vi "USUARIO_CONTRASENA.vi"(9 "INGRESAR (ENTER)":bool, 10 "Clave":string, 11 "Nombre":string) -> (1 "String 2":string, 2 "ACCESO":bool)   [LabVIEW 2019, in "HMI Class 3.lvclass"]
uses:
  HMI Class 3.lvclass
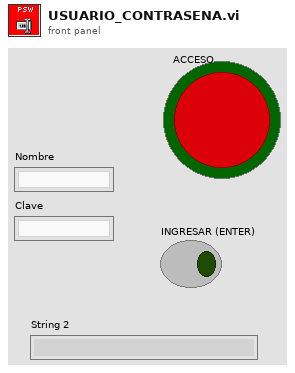
[diagram p1: front panel]
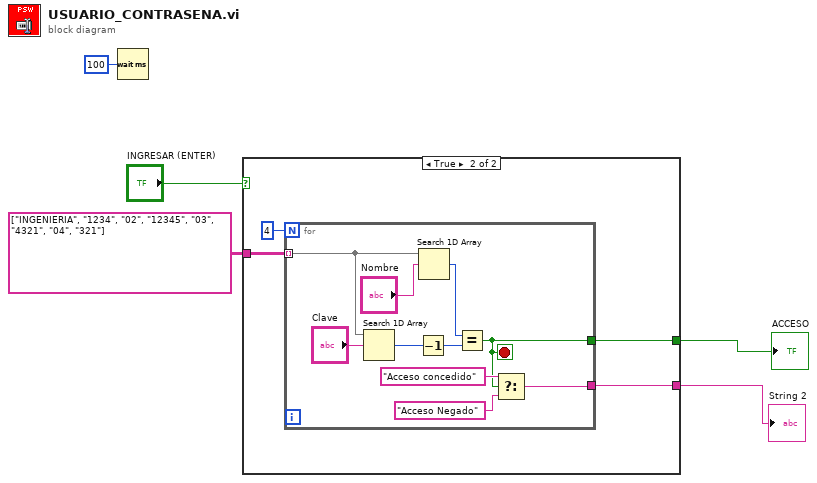
[diagram p0: block diagram]
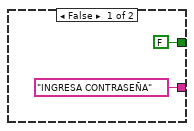
[diagram p2: hidden frame]
diagram:
  n1 = Wait (ms)(milliseconds to wait=u32 100) -> ()  [unwired: 1 out]
  n2 = case shown="True" "INGRESAR (ENTER)" {
    tunnel: string[][] [["INGENIERIA", "1234"], ["02", "12345"], ["03", "4321"], ["04", "321"]] -> [_ w11]
    tunnel: [FALSE w9] -> w3
    tunnel: ["INGRESA CONTRASEÑA" ("y") w8] -> w2
    frame False {
    }
    frame True {
      n3 = for {
        N: 4 -> [_]
        tunnel: w11 -> [w18] mode=indexing
        tunnel: [w13] -> w9
        tunnel: [w12] -> w8
        stop <- w13 stop-if-true
        n4 = Search 1D Array(1D array=w18, element="Clave") -> (index of element=w16:i32)  [unwired: 1 in]
        n5 = Decrement(x=w16) -> (x-1=w14:i32)
        n6 = Search 1D Array(1D array=w18, element="Nombre") -> (index of element=w15:i32)  [unwired: 1 in]
        n7 = Equal?(x=w15, y=w14) -> (x = y?=w13:bool)
        n8 = Select(t="Acceso concedido" ("y"), s=w13, f="Acceso Negado" ("y")) -> (s? t:f=w12:string)
      }
    }
  }
  "ACCESO" <- w3
  "String 2" <- w2
